vi "Get Array Elements.vi"(6 "Pass non-arrays":bool, 8 "error in (no error)":errorcluster, 10 "Offset":i32, 11 "JSON":string) -> (0 "error out":errorcluster, 1 "<JSON>":string[](array[string]) caption="<JSON>Elements", 2 "Offset past":i32 caption="Offset past Array")   [LabVIEW 2024, in "JSONtext.lvlib"]
doc: "If a JSON Array, returns all elements of the Array.\n\nIf the input JSON is not an Array, this function will return an error, unless \"Pass non-arrays\" is true, in which case the output will be a one-element array containing the input JSON."
uses:
  JSONtext.lvlib
  Parsing State.ctl
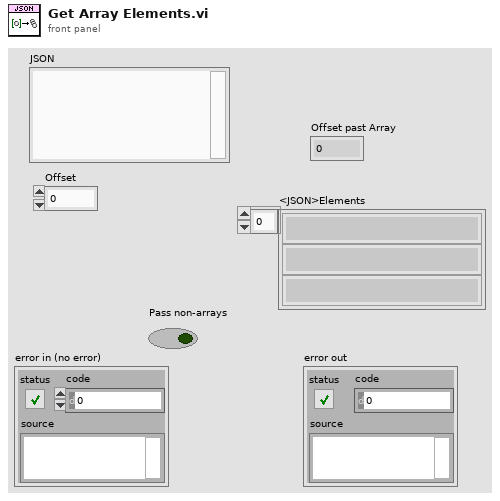
[diagram p1: front panel]
types:
  T1 = typedef "JSONtext.lvlib/Parsing State.ctl" = enum16{"Parser Error", "Object", "Array", "String", "Number/Other", "Leading Whitespace", "Object end", "Array end", "Value end"}
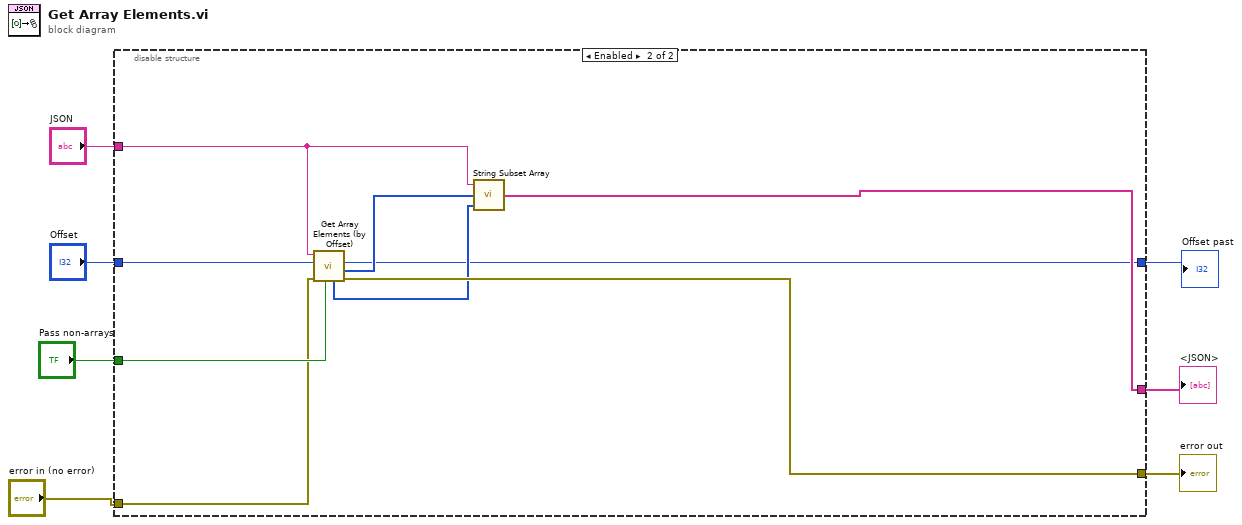
[diagram p0: block diagram]
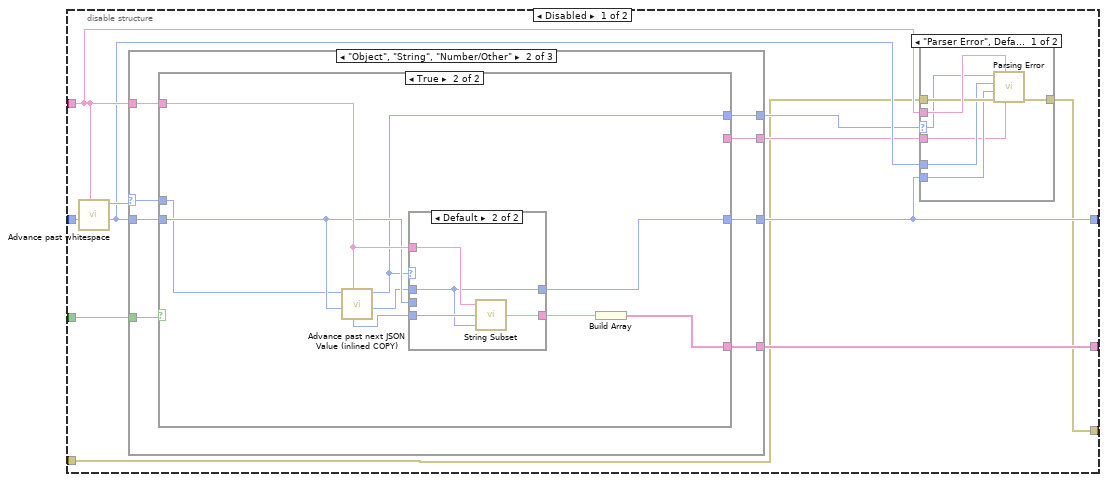
[diagram p2: hidden frame]
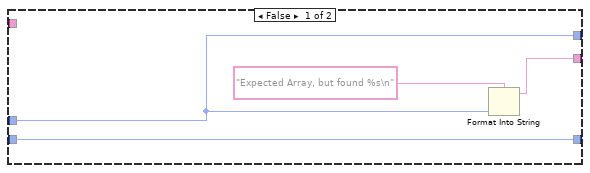
[diagram p5: hidden frame]
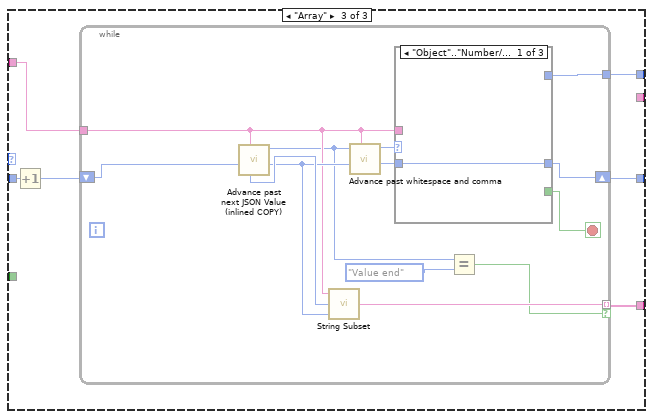
[diagram p7: hidden frame]
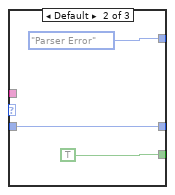
[diagram p8: hidden frame]
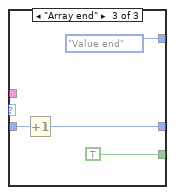
[diagram p9: hidden frame]
diagram:
  n1 = disable-structure shown="Enabled" {
    disable-tunnel: [w18 w83] -> w7
    disable-tunnel: "Offset" -> [w17 w90]
    disable-tunnel: "JSON" -> [w15 w86]
    disable-tunnel: [w13 w82] -> w4
    disable-tunnel: [w12 w87] -> w3
    disable-tunnel: "Pass non-arrays" -> [w10 w89]
    disable-tunnel: "error in (no error)" -> [w8 w88]
    frame Disabled {
      n2 = call "Advance past whitespace.vi"("JSON"=w15, "Offset"=w17) -> ("Offset of first non-whitespace"=w14:i32, "Parser State"=w16:T1)  [unwired: 7 in, 1 out]
      n3 = case shown="\"Object\", \"String\", \"Number/Other\"" w16 {
        selector: w16 -> [w28 w30 _]
        tunnel: [w28 w32 w60] -> w11
        tunnel: [w27 w33 w59] -> w13
        tunnel: [_ w34 w57] -> w18
        tunnel: w15 -> [_ w36 w56]
        tunnel: w14 -> [w27 w35 w55]
        tunnel: w10 -> [_ w31 _]
        tunnel: [_ w29 _] -> w9
        frame "Parser Error", Default {
        }
        frame "Object", "String", "Number/Other" {
          n4 = case shown="True" w31 {
            tunnel: w36 -> [_ w49]
            tunnel: w35 -> [w40 w48]
            tunnel: [_ w44] -> w34
            tunnel: [w40 w43] -> w33
            tunnel: [w38 w42] -> w32
            tunnel: w30 -> [w38 w41]
            tunnel: [w37 _] -> w29
            frame False {
              n5 = Format Into String(format string="Expected Array, but found %s\n", w38) -> (resulting string=w37:string)  [unwired: 2 in, 1 out]
            }
            frame True {
              n6 = call "Advance past next JSON Value (inlined COPY).vi"("JSON"=w49, "Offset"=w48, "State"=w41) -> ("Offset"=w47:i32, "State"=w42:T1, "Value start"=w46:i32)  [unwired: 4 in, 2 out]
              n7 = case shown="Default" w42 {
                tunnel: w46 -> [_ w54]
                tunnel: w48 -> [_ _]
                tunnel: w47 -> [w50 w51]
                tunnel: [_ w53] -> w45
                tunnel: w49 -> [_ w52]
                tunnel: [w50 w51] -> w43
                frame "Parser Error" {
                }
                frame Default {
                  n8 = call "String Subset.vi"("Offset past End"=w51, "Start offset"=w54, "JSON"=w52) -> ("substring"=w53:string)  [unwired: 2 in]
                }
              }
              n9 = Build Array(w45) -> (w44:string[])
            }
          }
        }
        frame "Array" {
          n10 = Increment(x=w55) -> (x+1=w58:i32)
          n11 = while {
            tunnel: w56 -> [w65]
            shift-right: [w70] -> w59
            shift-left: w58 -> [w71]
            tunnel: [w68] -> w60
            tunnel: [w62] -> w57 mode=indexing if=w61
            stop <- w69 stop-if-true
            n12 = call "Advance past next JSON Value (inlined COPY).vi"("JSON"=w65, "Offset"=w71) -> ("Offset"=w66:i32, "State"=w63:T1, "Value start"=w67:i32)  [unwired: 5 in, 2 out]
            n13 = call "String Subset.vi"("Offset past End"=w66, "Start offset"=w67, "JSON"=w65) -> ("substring"=w62:string)  [unwired: 2 in]
            n14 = call "Advance past whitespace and comma.vi"("JSON"=w65, "Offset"=w66, "State in"=w63) -> ("Offset past match"=w73:i32, "State"=w72:T1)  [unwired: 6 in, 1 out]
            n15 = case shown="\"Object\"..\"Number/Other\"" w72 {
              tunnel: [_ TRUE TRUE] -> w69
              tunnel: [_ Parsing_State."Parser Error" Parsing_State."Value end"] -> w68
              tunnel: w73 -> [w74 w75 w79]
              tunnel: [w74 w75 w78] -> w70
              tunnel: w65 -> [_ _ _]
              frame "Object".."Number/Other" {
              }
              frame Default {
              }
              frame "Array end" {
                n16 = Increment(x=w79) -> (x+1=w78:i32)
              }
            }
            n17 = Equal?(x=w63, y=Parsing_State."Value end") -> (x = y?=w61:bool)
          }
        }
      }
      n18 = case shown="\"Parser Error\", Default" w11 {
        selector: w11 -> [w20 _]
        tunnel: w15 -> [w25 _]
        tunnel: w8 -> [w24 w26]
        tunnel: [w23 w26] -> w12
        tunnel: w14 -> [w22 _]
        tunnel: w13 -> [w21 _]
        tunnel: w9 -> [w19 _]
        frame "Parser Error", Default {
          n19 = call "Parsing Error.vi"("initial string"=w19, "JSON"=w25, "error in (no error)"=w24, "Offset past match"=w21, "Value start"=w22, "State"=w20) -> ("error out"=w23:errorcluster)  [unwired: 5 in]
        }
        frame "Value end" {
        }
      }
    }
    frame Enabled {
      n20 = call "Get Array Elements (by Offset).vi"("Pass non-arrays"=w89, "error in (no error)"=w88, "Offset"=w90, "JSON"=w86) -> ("error out"=w87:errorcluster, "Element Offsets"=w85:i32[], "Offset past"=w82:i32, "Element End Offsets"=w84:i32[])  [unwired: 4 in]
      n21 = call "String Subset Array.vi"("Offset past End"=w84, "Start offset"=w85, "JSON"=w86) -> ("Subsets"=w83:string[])  [unwired: 2 in]
    }
  }
  "Offset past" <- w4
  "<JSON>" <- w7
  "error out" <- w3
